vi "DeCoF flush buffer.vi"(4 "error in (no error)":errorcluster, 7 "Connection ID in":T1) -> (0 "error out":errorcluster, 2 "read buffer":string, 3 "Conncection ID out":T1)   [LabVIEW 2013]
doc: "Flushes the input buffer of the remote connection."
uses:
  DeCoF connection.ctl
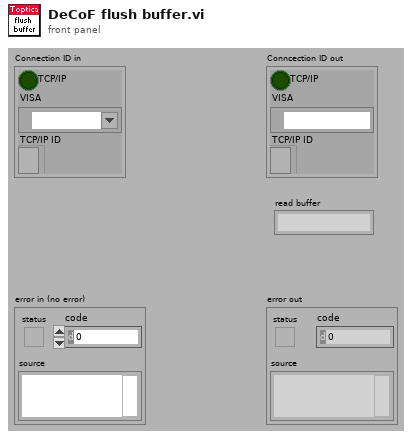
[diagram p1: front panel]
types:
  T1 = typedef "DeCoF connection.ctl" = cluster{"TCP/IP":bool, "VISA":refnum<visa-resource-name>, "TCP/IP ID":refnum<k5>}
  T2 = enum16{"Standard", "Buffered", "CRLF", "Immediate"}
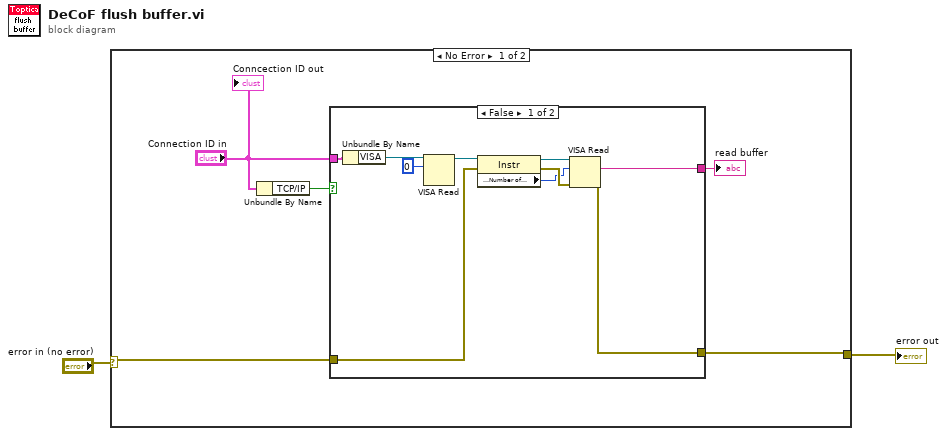
[diagram p0: block diagram]
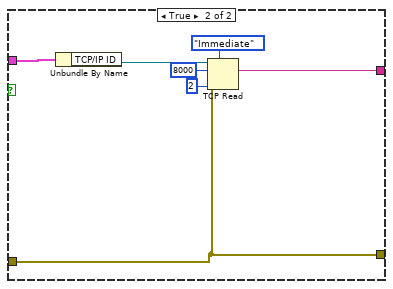
[diagram p2: hidden frame]
diagram:
  n1 = case shown="No Error" "error in (no error)" {
    selector: "error in (no error)" -> [w7 w25]
    tunnel: [w6 w25] -> w1
    frame No Error {
      n2 = Unbundle By Name("Connection ID in") -> ("TCP/IP"=w3:bool)
      n3 = case shown="False" w3 {
        tunnel: "Connection ID in" -> [w9 w20]
        tunnel: w7 -> [w15 w22]
        tunnel: [w11 w22] -> w6
        tunnel: [w10 w21] -> w5
        frame False {
          n4 = Unbundle By Name(w9) -> ("VISA"=w8:refnum<visa-resource-name>)
          n5 = VISA Read(VISA resource name=w8, byte count=u32 0) -> (VISA resource name out=w16:refnum<visa-resource-name>)  [unwired: 1 in, 3 out]
          n6 = property class="Instr"(reference=w16, error in=w15) -> (reference out=w13:refnum<visa-resource-name>, error out=w14:errorcluster, "Serial Settings:Number of Bytes at Serial Port"=w12:u32)
          n7 = VISA Read(VISA resource name=w13, byte count=w12, error in (no error)=w14) -> (read buffer=w10:string, error out=w11:errorcluster)  [unwired: 2 out]
        }
        frame True {
          n8 = Unbundle By Name(w20) -> ("TCP/IP ID"=w19:refnum<k5>)
          n9 = TCP Read(connection ID=w19, bytes to read=8000, error in (no error)=w22, 7:T2."Immediate" ("mode (standard)"), 9:2 ("timeout ms (25000)")) -> (data out=w21:string)  [unwired: 2 out]
        }
      }
      "read buffer" <- w5
      "Conncection ID out" <- "Connection ID in"
    }
    frame Error {
    }
  }
  "error out" <- w1
